vi "test 3-icon-demo-2-simple.vi"() -> ()   [LabVIEW 2019]
uses:
  _ctrl/BP4610_config.ctl
  _ctrl/rw.ctl
  _ctrl/BP4610_cmd.ctl
panel:
  in  "BP4610 Config":T1={"VISA"="", "Limit-BP"={"Set"=enum."Current", "Voltage+[V]"=20.0, "Current+[A]"=5.0, "Voltage-[V]"=-20.0, "Current-[A]"=-5.0}, "SET BP"={"Set"=enum."FREQ/WAVE", "Operation mode"=0, "Voltage[Vp-p]"=0.0, "Current[Ap-p]"=0.0, "Voltage[V]"=0.0, "Current[A]"=0.0, "Frequency[Hz]"=1.0, "Waveform"=enum."Sine"}} {"SET BP"."Frequency[Hz]" min=1.0 max=100000.0 step=0.1; "SET BP"."Current[A]" min=-20.0 max=20.0 step=0.001; "SET BP"."Voltage[V]" min=-115.0 max=115.0 step=0.01; "SET BP"."Current[Ap-p]" min=0.0 max=60.0 step=0.01; "SET BP"."Voltage[Vp-p]" min=0.0 max=120.0 step=0.1; "SET BP"."Operation mode" items=["CV-INT", "CV-EXT", "CV-ADD", "CC-INT", "CC-EXT", "CC-ADD"]; "Limit-BP"."Current-[A]" min=-20.0 max=20.0 step=0.001; "Limit-BP"."Voltage-[V]" min=-115.0 max=115.0 step=0.01; "Limit-BP"."Current+[A]" min=0.0 max=60.0 step=0.01; "Limit-BP"."Voltage+[V]" min=0.0 max=120.0 step=0.1}
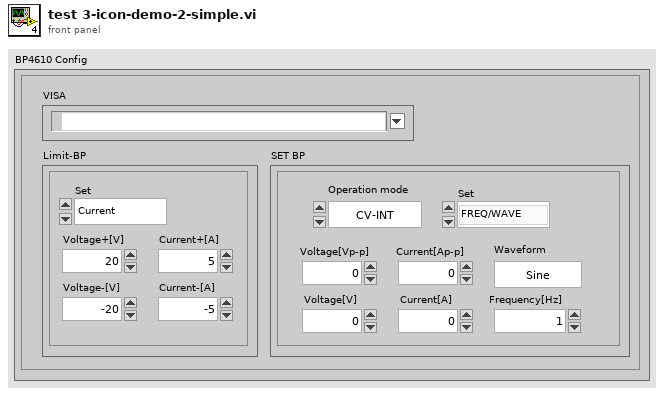
[diagram p1: front panel]
types:
  T1 = typedef "BP4610_config.ctl" = cluster{"VISA":refnum<visa-resource-name>, "Limit-BP":cluster{"Set":enum16{"Current", "Voltage"}, "Voltage+[V]":dbl, "Current+[A]":dbl, "Voltage-[V]":dbl, "Current-[A]":dbl}, "SET BP":cluster{"Set":enum16{"Current", "Voltage", "FREQ/WAVE"}, "Operation mode":u16, "Voltage[Vp-p]":dbl, "Current[Ap-p]":dbl, "Voltage[V]":dbl, "Current[A]":dbl, "Frequency[Hz]":dbl, "Waveform":enum16{"Sine", "Square", "ARB 1", "ARB 2", "ARB 3", "ARB 4", "ARB 5", "ARB 6", "ARB 7", "ARB 8", "ARB 9", "ARB 10", "ARB 11", "ARB 12", "ARB 13", "ARB 14", "ARB 15", "ARB 16"}}}
  T2 = typedef "rw.ctl" = enum16{"read", "write"}
  T3 = typedef "BP4610_cmd.ctl" = enum16{"open", "read", "set", "limit", "output on", "output off", "close"}
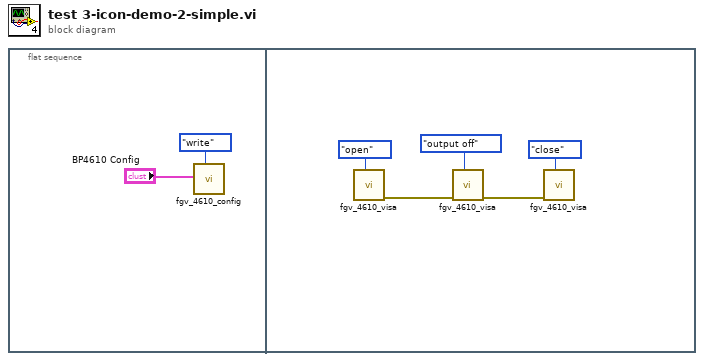
[diagram p0: block diagram]
diagram:
  n1 = flat-sequence {
    frame #0 {
      n2 = call "fgv_4610_config.vi"("cmd"=rw."write", "BP4610 Config"="BP4610 Config") -> ()  [unwired: 8 in, 2 out]
    }
    frame #1 {
      n3 = call "fgv_4610_visa.vi"("cmd"=BP4610_cmd."open") -> ("error out"=w4:errorcluster)  [unwired: 10 in]
      n4 = call "fgv_4610_visa.vi"("cmd"=BP4610_cmd."output off", "error in"=w4) -> ("error out"=w5:errorcluster)  [unwired: 9 in]
      n5 = call "fgv_4610_visa.vi"("cmd"=BP4610_cmd."close", "error in"=w5) -> ()  [unwired: 9 in, 1 out]
    }
  }
